vi "Compile UEGO.vi"(8 "error in (no error)":errorcluster, 10 "PB-01 Compiled Data":T1, 11 "Device Item Ref in":T4 format="%.0x") -> (0 "error out":errorcluster, 2 "PB-01 Compiled Data out":T1, 3 "Device Item Ref out":T4 format="%.0x")   [LabVIEW 2015, in "DCM System Explorer.lvlib"]
uses:
  DCM System Explorer.lvlib
  <vilib>/NI Veristand/Custom Device API/Custom Device Item Ref.ctl
  Shared/Types/PB-01.ctl
  Shared/Types/ESTTL Setup Indexes.ctl
  <vilib>/Powertrain Controls/Device Drivers/VR-Hall/RevC/Real-Time/Support/Vr_Hall_mode_control_revc.ctl
  Shared/DCM Constants and GUIDs.vi
  <vilib>/NI Veristand/Custom Device Tools/Custom Device Utility Library/NI VeriStand - Search for Item by GUID.vi
  <vilib>/NI Veristand/Custom Device Tools/Custom Device Utility Library/Custom Device Utility Library.lvlib
  DCM Shared.lvlib
  <vilib>/NI VeriStand/Custom Device API/Custom Device API.lvlib
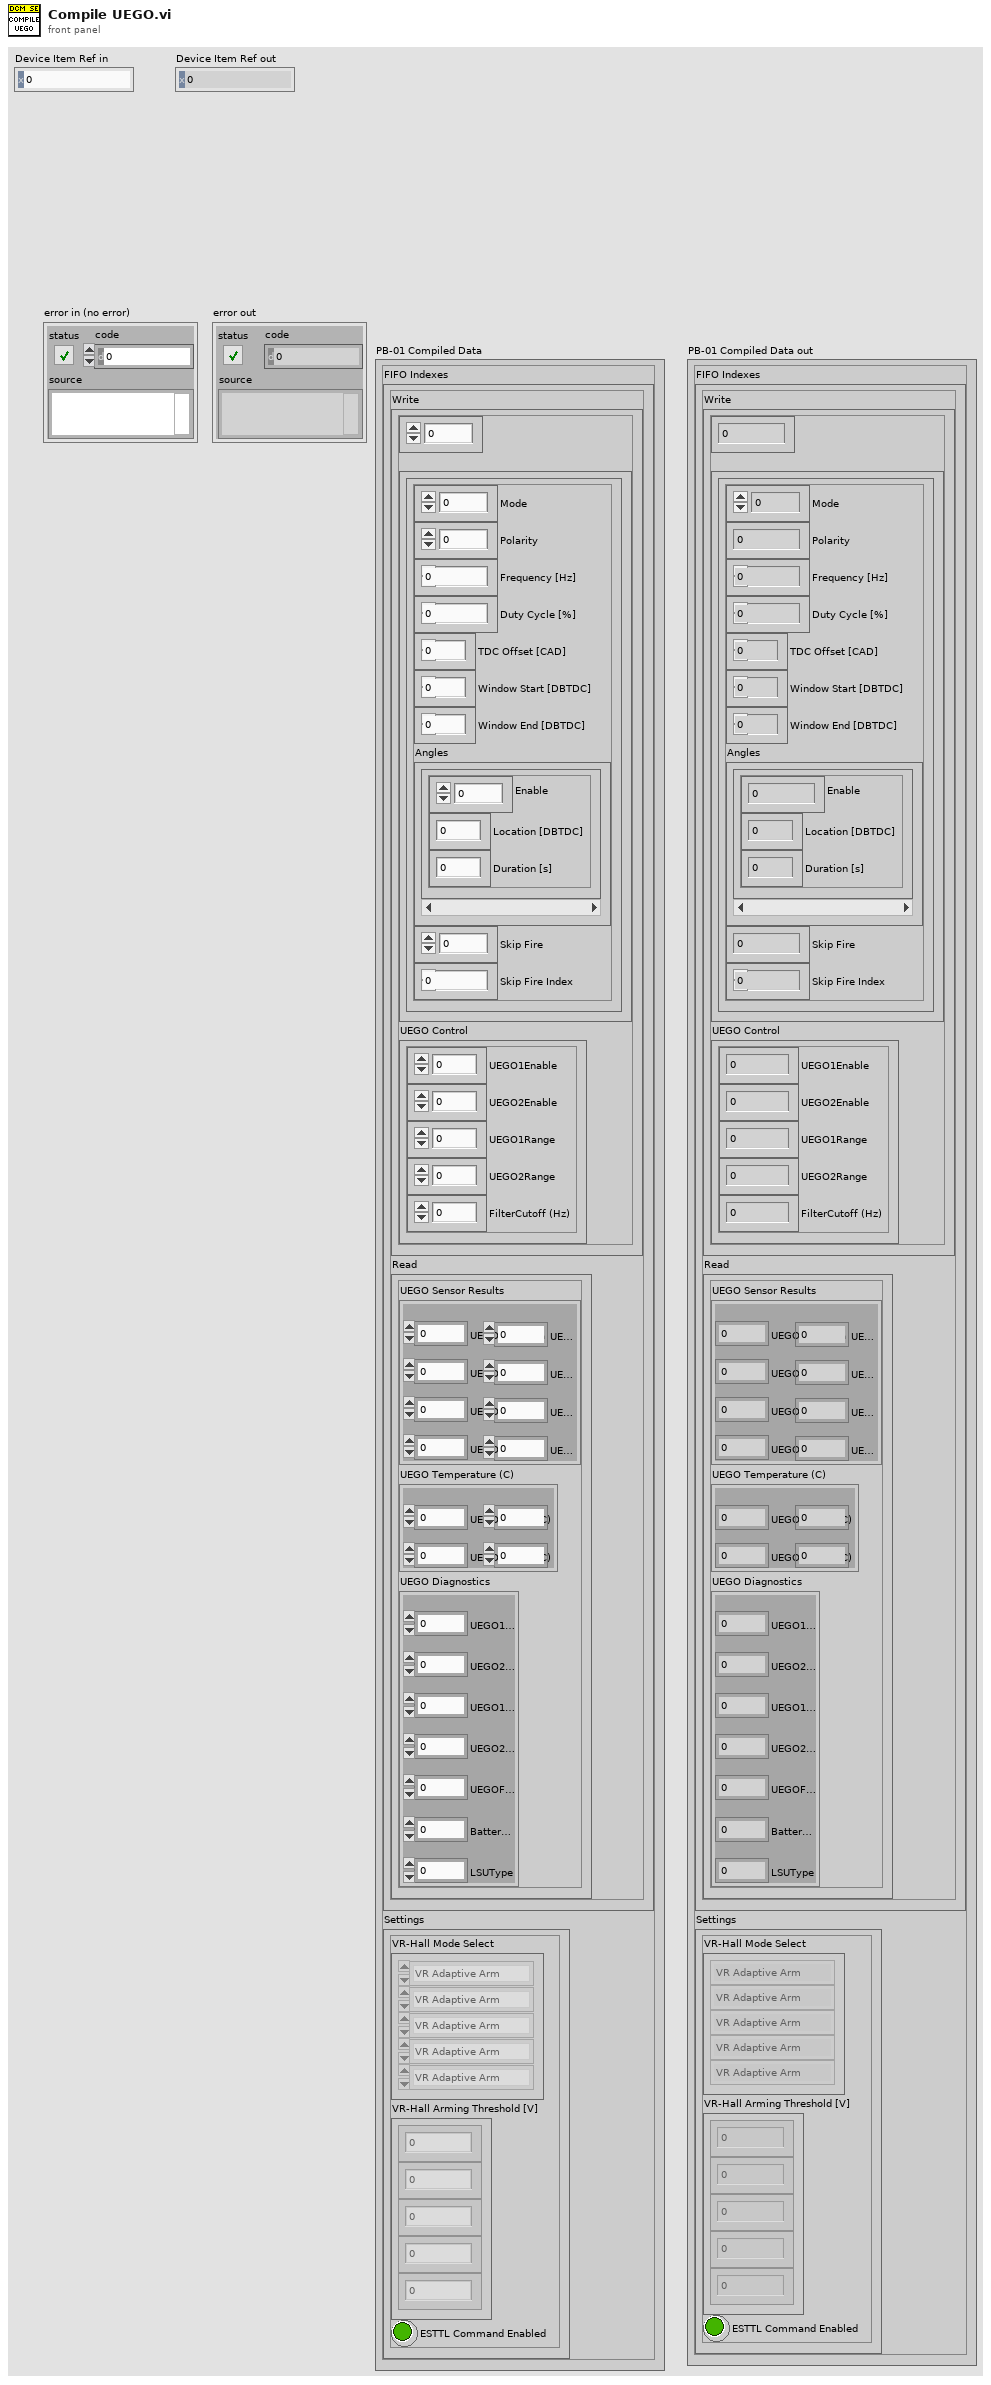
[diagram p1: front panel]
types:
  T1 = typedef "DCM Shared.lvlib/PB-01.ctl" = cluster{"FIFO Indexes":cluster{"Write":cluster{"Clear Faults":i32, "ESTTL Setup":T2[], "UEGO Control":cluster{"UEGO1Enable":i32, "UEGO2Enable":i32, "UEGO1Range":i32, "UEGO2Range":i32, "FilterCutoff (Hz)":i32}}, "Read":cluster{"UEGO Sensor Results":cluster{"UEGO1Lambda":i32, "UEGO1Phi":i32, "UEGO1AFRatio":i32, "UEGO1Ip (mA)":i32, "UEGO2Lambda":i32, "UEGO2Phi":i32, "UEGO2AFRatio":i32, "UEGO2Ip (mA)":i32}, "UEGO Temperature (C)":cluster{"UEGO1Temp (C)":i32, "UEGO2Temp (C)":i32, "UEGO1Hot":i32, "UEGO2Hot":i32}, "UEGO Diagnostics":cluster{"UEGO1SensorFault":i32, "UEGO2SensorFault":i32, "UEGO1HeaterFault":i32, "UEGO2HeaterFault":i32, "UEGOFuseStatus":i32, "Battery (V)":i32, "LSUType":i32}}}, "Settings":cluster{"VR-Hall Mode Select":T3[], "VR-Hall Arming Threshold [V]":dbl[], "ESTTL Command Enabled":bool}}
  T2 = typedef "DCM Shared.lvlib/ESTTL Setup Indexes.ctl" = cluster{"Mode":i32, "Polarity":i32, "Frequency [Hz]":i32, "Duty Cycle [%]":i32, "TDC Offset [CAD]":i32, "Window Start [DBTDC]":i32, "Window End [DBTDC]":i32, "Angles":cluster{"Enable":i32, "Location [DBTDC]":i32, "Duration [s]":i32}[], "Skip Fire":i32, "Skip Fire Index":i32}
  T3 = typedef "Vr_Hall_mode_control_revc.ctl" = enum32{"VR Adaptive Arm", "VR Manual Arm", "Hall", "Hall w/ Pull-up"}
  T4 = typedef "Custom Device API.lvlib/Custom Device Item Ref.ctl" = u64
  T5 = typedef "DCM Shared.lvlib/Channel.ctl" = cluster{"Name":string, "Units":string, "Default":dbl, "Description":string}
  T6 = cluster{"FIFO indexes[0]":i32, "FIFO indexes[1]":i32, "FIFO indexes[2]":i32, "FIFO indexes[3]":i32, "FIFO indexes[4]":i32}
  T7 = cluster{"FIFO indexes[0]":i32, "FIFO indexes[1]":i32, "FIFO indexes[2]":i32, "FIFO indexes[3]":i32, "FIFO indexes[4]":i32, "FIFO indexes[5]":i32, "FIFO indexes[6]":i32, "FIFO indexes[7]":i32}
  T8 = cluster{"FIFO indexes[0]":i32, "FIFO indexes[1]":i32, "FIFO indexes[2]":i32, "FIFO indexes[3]":i32}
  T9 = cluster{"FIFO indexes[0]":i32, "FIFO indexes[1]":i32, "FIFO indexes[2]":i32, "FIFO indexes[3]":i32, "FIFO indexes[4]":i32, "FIFO indexes[5]":i32, "FIFO indexes[6]":i32}
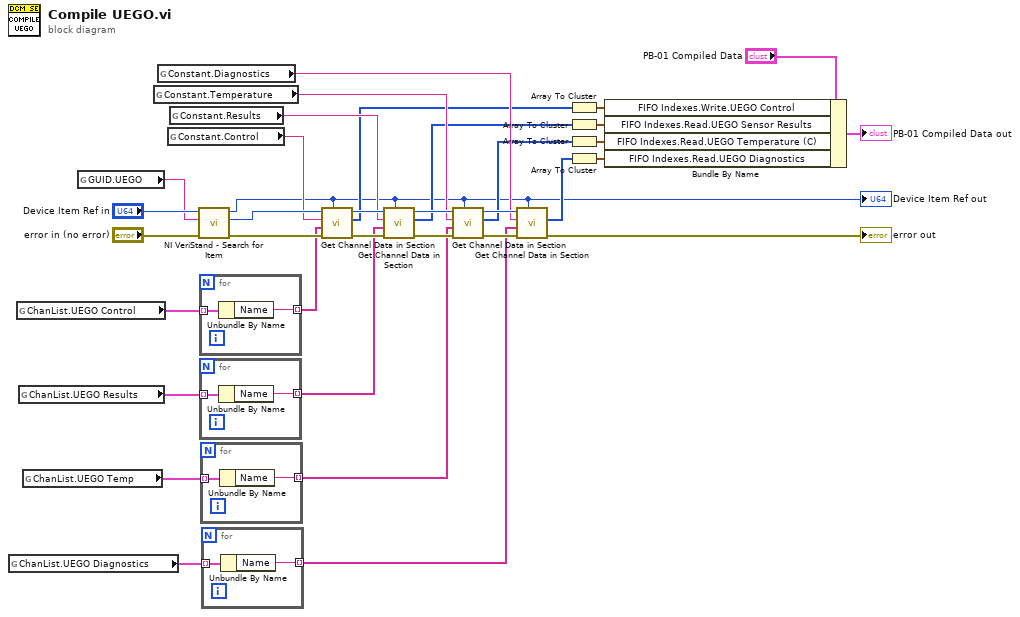
[diagram p0: block diagram]
diagram:
  n1 = global read "DCM Constants and GUIDs.vi" "ChanList.UEGO Diagnostics"() -> (w19:T5[])
  n2 = global read "DCM Constants and GUIDs.vi" "ChanList.UEGO Control"() -> (w20:T5[])
  n3 = global read "DCM Constants and GUIDs.vi" "ChanList.UEGO Results"() -> (w21:T5[])
  n4 = global read "DCM Constants and GUIDs.vi" "ChanList.UEGO Temp"() -> (w22:T5[])
  n5 = global read "DCM Constants and GUIDs.vi" "GUID.UEGO"() -> (w33:string)
  n6 = global read "DCM Constants and GUIDs.vi" "Constant.Temperature"() -> (w12:string)
  n7 = global read "DCM Constants and GUIDs.vi" "Constant.Diagnostics"() -> (w13:string)
  n8 = global read "DCM Constants and GUIDs.vi" "Constant.Control"() -> (w17:string)
  n9 = global read "DCM Constants and GUIDs.vi" "Constant.Results"() -> (w11:string)
  n10 = call-poly <vilib>:"NI VeriStand - Search for Item.vi"("error in"="error in (no error)", "Item GUID"=w33, "Section Ref in"="Device Item Ref in") -> ("error out"=w29:errorcluster, "Item Ref"=w30:T4, "Section Ref out"=w1:T4)  [unwired: 5 in, 1 out]
  "Device Item Ref out" <- w1
  n11 = for {
    tunnel: w20 -> [w37] mode=indexing
    tunnel: [w36] -> w18 mode=indexing
    n12 = Unbundle By Name(w37) -> ("Name"=w36:string)
  }
  n13 = for {
    tunnel: w21 -> [w39] mode=indexing
    tunnel: [w38] -> w16 mode=indexing
    n14 = Unbundle By Name(w39) -> ("Name"=w38:string)
  }
  n15 = for {
    tunnel: w22 -> [w41] mode=indexing
    tunnel: [w40] -> w15 mode=indexing
    n16 = Unbundle By Name(w41) -> ("Name"=w40:string)
  }
  n17 = for {
    tunnel: w19 -> [w43] mode=indexing
    tunnel: [w42] -> w14 mode=indexing
    n18 = Unbundle By Name(w43) -> ("Name"=w42:string)
  }
  n19 = call "Get Channel Data in Section.vi"("Custom device ref"=w1, "error in (no error)"=w29, "Channels"=w18, "Section (\"\":none)"=w17, "Item Ref in"=w30) -> ("error out"=w28:errorcluster, "FIFO indexes"=w10:i32[], "Item Ref out"=w27:T4)  [unwired: 2 in, 2 out]
  n20 = call "Get Channel Data in Section.vi"("Custom device ref"=w1, "error in (no error)"=w28, "Channels"=w16, "Section (\"\":none)"=w11, "Item Ref in"=w27) -> ("error out"=w26:errorcluster, "FIFO indexes"=w7:i32[], "Item Ref out"=w25:T4)  [unwired: 2 in, 2 out]
  n21 = call "Get Channel Data in Section.vi"("Custom device ref"=w1, "error in (no error)"=w26, "Channels"=w15, "Section (\"\":none)"=w12, "Item Ref in"=w25) -> ("error out"=w24:errorcluster, "FIFO indexes"=w6:i32[], "Item Ref out"=w23:T4)  [unwired: 2 in, 2 out]
  n22 = call "Get Channel Data in Section.vi"("Custom device ref"=w1, "error in (no error)"=w24, "Channels"=w14, "Section (\"\":none)"=w13, "Item Ref in"=w23) -> ("error out"=→"error out":errorcluster, "FIFO indexes"=w5:i32[])  [unwired: 2 in, 3 out]
  n23 = Array To Cluster(array=w10) -> (cluster=w9:T6)
  n24 = Array To Cluster(array=w7) -> (cluster=w8:T7)
  n25 = Array To Cluster(array=w6) -> (cluster=w4:T8)
  n26 = Array To Cluster(array=w5) -> (cluster=w3:T9)
  n27 = Bundle By Name(cluster="PB-01 Compiled Data", "FIFO Indexes.Write.UEGO Control"=w9, "FIFO Indexes.Read.UEGO Sensor Results"=w8, "FIFO Indexes.Read.UEGO Temperature (C)"=w4, "FIFO Indexes.Read.UEGO Diagnostics"=w3) -> (→"PB-01 Compiled Data out":T1)
